vi "Test Dummy VI.vi"(8 "Error In":errorcluster) -> (0 "Error Out":errorcluster, 3 "Array":dbl[](array[numeric]))   [LabVIEW 2014]
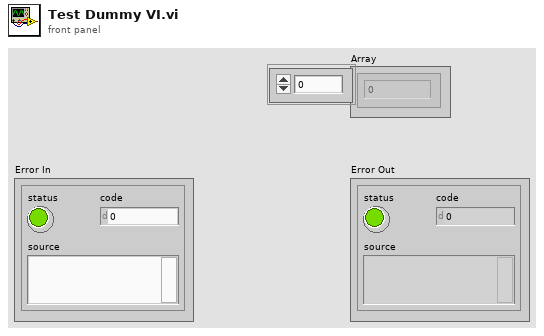
[diagram p1: front panel]
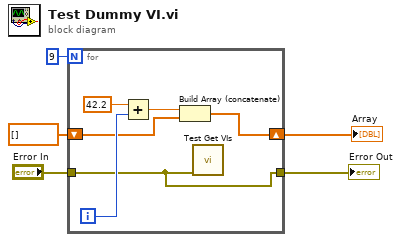
[diagram p0: block diagram]
diagram:
  n1 = for {
    N: 9 -> [_]
    tunnel: [w6] -> w5
    tunnel: "Error In" -> [w6]
    shift-right: [w8] -> w3
    shift-left: dbl[] [] -> [w7]
    i -> [w9]
    n2 = Add(x=42.2, y=w9) -> (x+y=w10:dbl)
    n3 = Build Array (concatenate)(w10, w7) -> (w8:dbl[])
    n4 = call "Test Get VIs.vi"("Error In"=w6) -> ()  [unwired: 11 in]
  }
  "Error Out" <- w5
  "Array" <- w3
